vi "chart series set values lv.vi"(5 "last_col":u16, 6 "last_row":u32, 7 "first_col":u16, 8 "error in (no error)":errorcluster, 9 "first_row":u32, 10 "sheetname":string, 11 "series":u32) -> (0 "error out":errorcluster)   [LabVIEW 8.6]
doc: "void chart_series_set_values_lv(lxw_chart_series series, const char *sheetname, lxw_row_t first_row, lxw_col_t first_col, lxw_row_t last_row, lxw_col_t last_col);"
uses:
  pending_lvxlsxwriter/xlsxwriter.dll
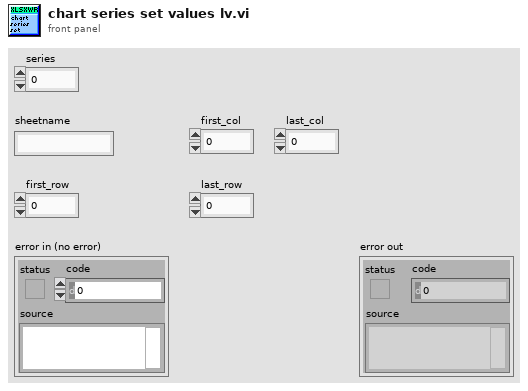
[diagram p1: front panel]
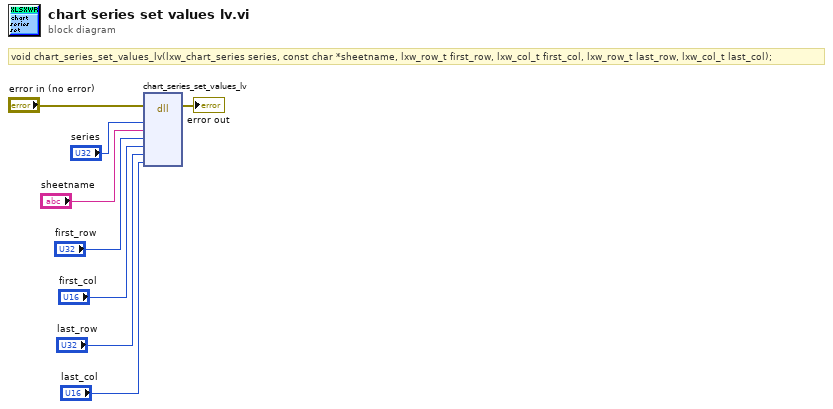
[diagram p0: block diagram]
diagram:
  # "void chart_series_set_values_lv(lxw_chart_series series, const char *sheetname, lxw_row_t first_row, lxw_col_t first_col, lxw_row_t last_row, lxw_col_t last_col);"
  n1 = dll-call lib="C:/Users/WDAGUtilityAccount/Desktop/pending_lvxlsxwriter/xlsxwriter.*" fn="chart_series_set_values_lv"(error in="error in (no error)", "series"="series", "sheetname"="sheetname", "first_row"="first_row", "first_col"="first_col", "last_row"="last_row", "last_col"="last_col") -> (error out=→"error out":errorcluster)  [unwired: 9 in, 1 out]
